vi "PRUEBA_CALIBRACION.vi"() -> ()   [LabVIEW 2015]
doc: "This VI reads a buffer of single point values from all four channels of the NI 923x and places the acquired data into a DMA FIFO."
uses:
  <vilib>/eio/EIOPropertyNode/EIOPropertyNode.xnode
  <vilib>/eio/EIONode/EIONode.xnode
  <vilib>/rvi/DataTransferAndStorage/Container/XNode/niFpgaContainer.xnode
  <vilib>/rvi/eio/common/nirviEmuTemplateMethod_errors.vi
  <vilib>/LabVIEW Targets/FPGA/cRIO/shared/nicrio_ModuleControls/nicrio_cRIO-9234_DataRatesRing2.ctl
  <vilib>/rvi/eio/common/nirviEmuTemplatePropertyGet_errors.vi
  <vilib>/rvi/eio/common/nirviEmuTemplatePropertyGet_noerrors.vi
  <vilib>/rvi/eio/common/nirviEmuTemplatePropertySet_errors.vi
  <vilib>/rvi/eio/common/nirviEmuTemplatePropertySet_noerrors.vi
  <vilib>/rvi/interface/RandomDataEmulation/nirviRandomDataFpgaReadWriteTemplate.vi
panel:
  out "appended array":fxp<+/-,24,4>[](array[numeric])
  out "Chassis Temperature":i16
  out "Fotocelula":bool
  out "Detector de\npresencia":bool
  in  "Fotocélula":bool
  out "DC OK":bool
  in  "Data Rate":T1=2 items=["51.200 kS/s (NI 9234)"=1, "25.600 kS/s (NI 9234)"=2, "17.067 kS/s (NI 9234)"=3, "12.800 kS/s (NI 9234)"=4, "10.240 kS/s (NI 9234)"=5, "8.533 kS/s (NI 9234)"=6, "7.314 kS/s (NI 9234)"=7, "6.400 kS/s (NI 9234)"=8, "5.689 kS/s (NI 9234)"=9, "5.120 kS/s (NI 9234)"=10, "4.654 kS/s (NI 9234)"=11, "4.267 kS/s (NI 9234)"=12, "3.938 kS/s (NI 9234)"=13, "3.657 kS/s (NI 9234)"=14, "3.413 kS/s (NI 9234)"=15, "3.200 kS/s (NI 9234)"=16, "3.012 kS/s (NI 9234)"=17, "2.845 kS/s (NI 9234)"=18, "2.695 kS/s (NI 9234)"=19, "2.560 kS/s (NI 9234)"=20, "2.438 kS/s (NI 9234)"=21, "2.328 kS/s (NI 9234)"=22, "2.226 kS/s (NI 9234)"=23, "2.133 kS/s (NI 9234)"=24, "2.048 kS/s (NI 9234)"=25, "1.969 kS/s (NI 9234)"=26, "1.896 kS/s (NI 9234)"=27, "1.829 kS/s (NI 9234)"=28, "1.765 kS/s (NI 9234)"=29, "1.707 kS/s (NI 9234)"=30, "1.652 kS/s (NI 9234)"=31]
  out "Buffer Overflow":bool
  in  "Stop":bool
  out "Buffer Underflow":bool
  out "Error Out":errorcluster
  # "For instructions, and select Help>>Show Context Help and hover over the icon."
  # "Timing Parameters"
  # "Output Parameters"
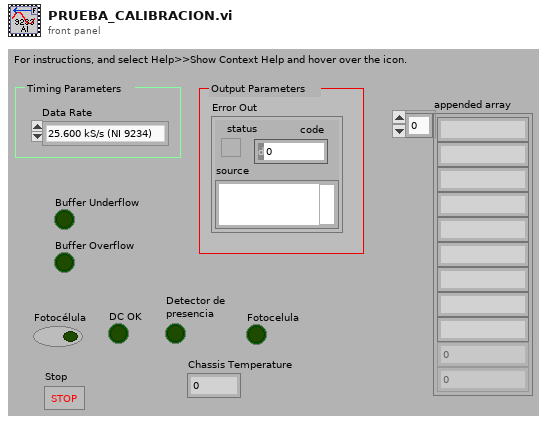
[diagram p1: front panel]
types:
  T1 = typedef "nicrio_cRIO-9234_DataRatesRing2.ctl" = u8
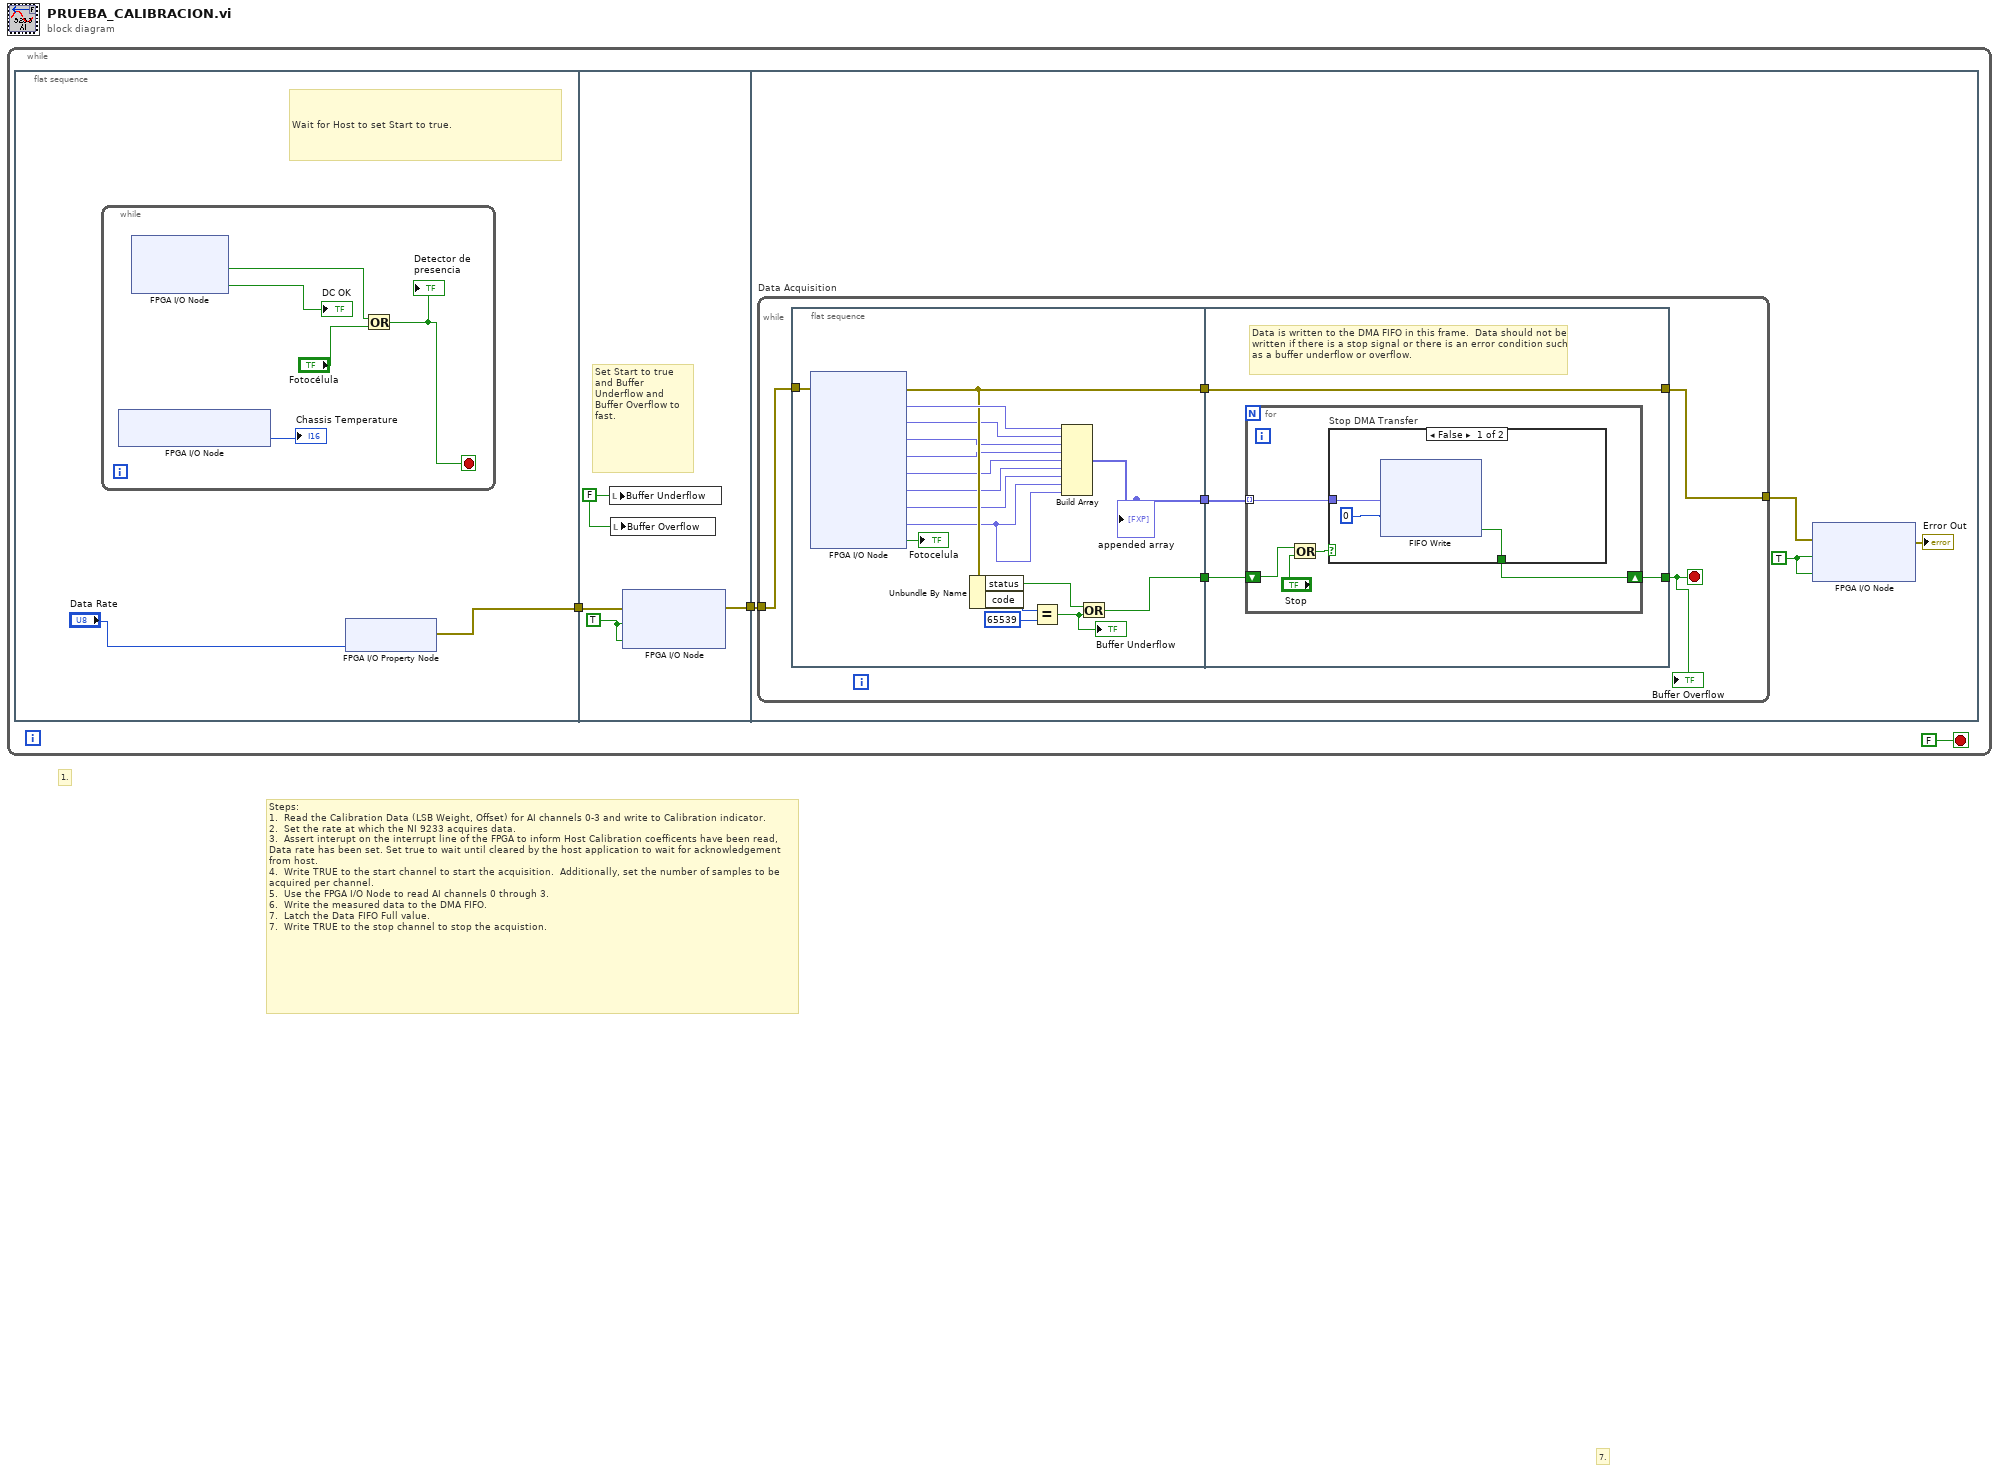
[diagram p0: block diagram]
diagram:
  # "7."
  # "Steps: \n1.  Read the Calibration Data (LSB Weight, Offset) for AI channels 0-3 and write to Calibration indicator.\n2.  Set the rate at which the NI 9233 acquires data. \n3.  Assert interupt on the interrupt line of the FPGA to inform Host Calibration coefficents have been read, Data rate has been set. Set true to wait until cleared by the host application to wait for acknowledgement from host.\n4.  Write TRUE to the start channel to start the acquisition.  Additionally, set the number of samples to be acquired per channel.\n5.  Use the FPGA I/O Node to read AI channels 0 through 3. \n6.  Write the measured data to the DMA FIFO.\n7.  Latch the Data FIFO Full value.\n7.  Write TRUE to the stop channel to stop the acquistion."
  # "1."
  n1 = while {
    stop <- FALSE stop-if-true
    n2 = flat-sequence "MainSeq" {
      tunnel: [w5] -> w2
      tunnel: w2 -> [w13]
      tunnel: [w12] -> w1
      tunnel: w1 -> [w18]
      frame #0 {
        # "Wait for Host to set Start to true."
        n3 = while "initWait" {
          stop <- w7 stop-if-true
          n4 = xnode "FPGA I/O Node"() -> ("Chassis Temperature"=→"Chassis Temperature":i16)  [unwired: 1 in, 1 out]
          n5 = xnode "FPGA I/O Node"() -> ("Mod3/DI0"=w9:bool, "Mod3/DI2"=→"DC OK":bool)  [unwired: 3 in, 3 out]
          n6 = Or(x=w9, y="Fotocélula") -> (x .or. y?=w7:bool)
          "Detector de\npresencia" <- w7
        }
        n7 = xnode "FPGA I/O Property Node"("Data Rate"="Data Rate") -> ("error out"=w5:errorcluster)  [unwired: 2 in, 1 out]
      }
      frame #1 {
        w11 = TRUE
        w14 = FALSE ("Late? (Latched)")
        # "Set Start to true and Buffer Underflow and Buffer Overflow to fast."
        n8 = local write "Buffer Underflow"(w14) -> ()
        n9 = local write "Buffer Overflow"(w14) -> ()
        n10 = xnode "FPGA I/O Node"("error in"=w13, "Mod1/Start"=w11, "Mod2/Start"=w11) -> ("error out"=w12:errorcluster)  [unwired: 2 in, 2 out]
      }
      frame #2 {
        w15 = TRUE
        n11 = while "Data Acquisition" {
          tunnel: w18 -> [w22]
          tunnel: [w21] -> w16
          stop <- w19 stop-if-true
          n12 = flat-sequence "Data Acquisition Sequence" {
            tunnel: [w40] -> w24
            tunnel: [w31] -> w23
            tunnel: w22 -> [w39]
            tunnel: [w38] -> w20
            tunnel: w24 -> [w45]
            tunnel: w23 -> [w44]
            tunnel: [w43] -> w19
            tunnel: [w42] -> w21
            tunnel: w20 -> [w42]
            frame #0 {
              n13 = xnode "FPGA I/O Node"("error in"=w39) -> ("error out"=w38:errorcluster, "Mod1/AI0"=w41:fxp<+/-,24,4>, "Mod1/AI1"=w34:fxp<+/-,24,4>, "Mod1/AI2"=w33:fxp<+/-,24,4>, "Mod1/AI3"=w32:fxp<+/-,24,4>, "Mod2/AI0"=w29:fxp<+/-,24,4>, "Mod2/AI1"=w28:fxp<+/-,24,4>, "Mod2/AI2"=w27:fxp<+/-,24,4>, "Mod2/AI3"=w25:fxp<+/-,24,4>, "Mod3/DI0"=→"Fotocelula":bool)  [unwired: 9 in, 9 out]
              n14 = Unbundle By Name(w38) -> ("status"=w30:bool, "code"=w37:i32)
              n15 = Equal?(x=w37, y=65539) -> (x = y?=w35:bool)
              "Buffer Underflow" <- w35
              n16 = Build Array(w41, w34, w33, w32, w29, w28, w27, w25, w25) -> (w40:fxp<+/-,24,4>[])
              "appended array" <- w40
              n17 = Or(x=w30, y=w35) -> (x .or. y?=w31:bool)
            }
            frame #1 {
              # "Data is written to the DMA FIFO in this frame.  Data should not be\nwritten if there is a stop signal or there is an error condition such \nas a buffer underflow or overflow."
              n18 = for "DMAWriteLoop" {
                tunnel: w45 -> [w50] mode=indexing
                shift-right: [w46] -> w43
                shift-left: w44 -> [w48]
                n19 = Or(x=w48, y="Stop") -> (x .or. y?=w47:bool)
                n20 = case "Stop DMA Transfer" shown="False" w47 {
                  selector: w47 -> [_ w54]
                  tunnel: w50 -> [w51 _]
                  tunnel: [w53 w54] -> w46
                  frame False {
                    n21 = xnode ("FIFO Write")("Element"=w51, "Timeout"=0) -> ("Timed Out?"=w53:bool)  [unwired: 1 in, 1 out]
                  }
                  frame True {
                  }
                }
              }
            }
          }
          "Buffer Overflow" <- w19
        }
        n22 = xnode "FPGA I/O Node"("error in"=w16, "Mod1/Stop"=w15, "Mod2/Stop"=w15) -> ("error out"=→"Error Out":errorcluster)  [unwired: 2 in, 2 out]
      }
    }
  }
